vi "SendCommand.vi"(0 "reference in":refnum<class "Redis.lvclass">, 7 "Command":string, 11 "Error In":errorcluster) -> (4 "reference out":refnum<class "Redis.lvclass">, 8 "Data":T1, 15 "Error Out":errorcluster)   [LabVIEW 2020, in "Redis.lvclass"]
uses:
  Redis.lvclass
  RedisDataType.ctl
  ReplyDataTypeEnum.ctl
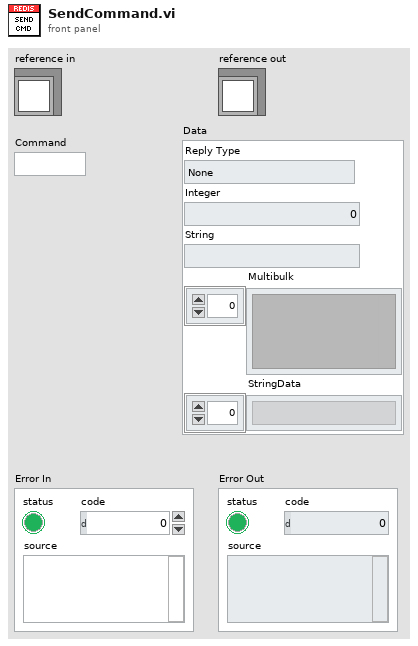
[diagram p1: front panel]
types:
  T1 = typedef "Redis.lvclass/RedisDataType.ctl" = cluster{"Reply Type":T2, "Integer":i64, "String":string, "Multibulk":variant[], "StringData":string[]}
  T2 = typedef "Redis.lvclass/ReplyDataTypeEnum.ctl" = enum16{"None", "Error", "Status", "Nil", "Integer", "String", "Multibulk"}
  T3 = typedef "Redis.lvclass/ObjectAttributes.ctl" = cluster{"Port":u32, "Host":string, "Username":string, "Password":string, "UseAuthentication":bool}
  T4 = typedef "Redis.lvclass/ReplyDataType.ctl" = cluster{"Integer":i64, "String":string, "Multibulk":variant[]}
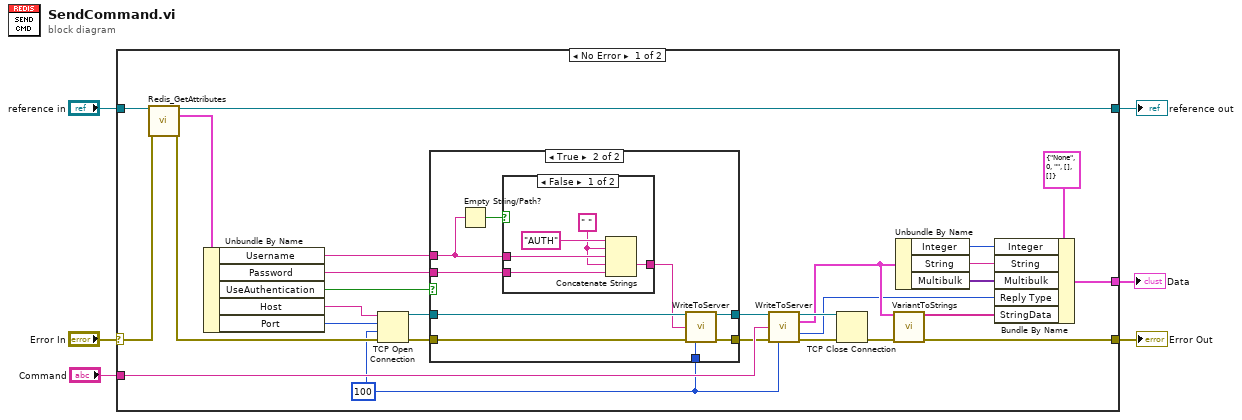
[diagram p0: block diagram]
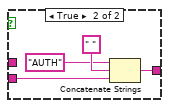
[diagram p3: hidden frame]
diagram:
  n1 = case shown="No Error" "Error In" {
    selector: "Error In" -> [w34 w56]
    tunnel: [w9 w56] -> w5
    tunnel: [w31 w55] -> w3
    tunnel: "reference in" -> [w32 w55]
    tunnel: "Command" -> [w25 _]
    tunnel: [w13 _] -> w1
    frame No Error {
      w20 = 100 ("timeout ms")
      n2 = call "Redis_GetAttributes.vi"("reference in"=w32, "Error In"=w34) -> ("reference out"=w31:refnum<class "Redis.lvclass">, "Data"=w33:T3, "Error Out"=w26:errorcluster)  [unwired: 10 in, 1 out]
      n3 = Unbundle By Name(w33) -> ("Username"=w18:string, "Password"=w17:string, "UseAuthentication"=w19:bool, "Host"=w28:string, "Port"=w27:u32)
      n4 = TCP Open Connection(address=w28, remote port or service name=w27, timeout ms (60000)=w20, error in (no error)=w26) -> (connection ID=w24:refnum<k5>, error out=w22:errorcluster)  [unwired: 1 in]
      n5 = case shown="True" w19 {
        tunnel: w24 -> [w36 w45]
        tunnel: [w36 w44] -> w23
        tunnel: w22 -> [w35 w43]
        tunnel: [w35 w42] -> w21
        tunnel: w20 -> [_ w41]
        tunnel: w18 -> [_ w39]
        tunnel: w17 -> [_ w38]
        frame False {
        }
        frame True {
          n6 = Empty String/Path?(string/path=w39) -> (empty?=w40:bool)
          n7 = case shown="False" w40 {
            tunnel: [w46 w53] -> w37
            tunnel: w38 -> [w48 w52]
            tunnel: w39 -> [w49 _]
            frame False {
              w47 = " "
              n8 = Concatenate Strings("AUTH", w47, w49, w47, w48) -> (w46:string)
            }
            frame True {
              n9 = Concatenate Strings("AUTH", " ", w52) -> (w53:string)
            }
          }
          n10 = call "WriteToServer.vi"("TCP in"=w45, "Command"=w37, "error in"=w43, "Timeout(1000ms)"=w41) -> ("TCP out"=w44:refnum<k5>, "error out"=w42:errorcluster)  [unwired: 8 in, 2 out]
        }
      }
      n11 = call "WriteToServer.vi"("TCP in"=w23, "Command"=w25, "error in"=w21, "Timeout(1000ms)"=w20) -> ("TCP out"=w29:refnum<k5>, "ReplyData"=w11:T4, "Reply Type"=w7:T2, "error out"=w30:errorcluster)  [unwired: 8 in]
      n12 = TCP Close Connection(connection ID=w29, error in (no error)=w30) -> (error out=w10:errorcluster)  [unwired: 1 in, 1 out]
      n13 = call "VariantToStrings.vi"("Data in"=w11, "error in"=w10) -> ("Strings"=w8:string[], "error out"=w9:errorcluster)  [unwired: 11 in, 1 out]
      n14 = Unbundle By Name(w11) -> ("Integer"=w14:i64, "String"=w15:string, "Multibulk"=w16:variant[])
      n15 = Bundle By Name(cluster=T1 {"Reply Type"=enum."None", "Integer"=0, "String"="", "Multibulk"=[], "StringData"=[]} ("Data"), "Integer"=w14, "String"=w15, "Multibulk"=w16, "Reply Type"=w7, "StringData"=w8) -> (w13:T1)
    }
    frame Error {
    }
  }
  "Error Out" <- w5
  "reference out" <- w3
  "Data" <- w1
